vi "background writer.vi"(0 "dictionary":T1, 1 "command queue":refnum<k33>, 2 "response from processor":refnum<k33>, 3 "output type order":T3[](array[typedef]), 5 "logging path":path, 7 "backup directory":path, 9 "cache allocation":T2, 11 "scans per write":u16=20, 12 "group name":string, 13 "enable channel (bool)":i32, 14 "has enable channel":bool) -> (15 "error out":errorcluster)   [LabVIEW 2013, in "TDMS datalogger runtime.lvclass"]
uses:
  TDMS datalogger runtime.lvclass
  <vilib>/NI/Tag Bus/tag/Data Type.ctl
  data cache.ctl
  <vilib>/NI/Tag Bus/dictionary/full data dictionary.ctl
  message to background process.ctl
  control enum.ctl
  <vilib>/NI/Tag Bus/table/data table.ctl
  response from background process.ctl
  response enum.ctl
  writer state enum.ctl
  move to cache.vi
  write cache to tdms.vi
  <vilib>/NI/Tag Bus/table/data table.lvlib
  <vilib>/NI/Tag Bus/tag/tag descriptor.lvclass
  <vilib>/NI/Tag Bus/dictionary/data dictionary.lvclass
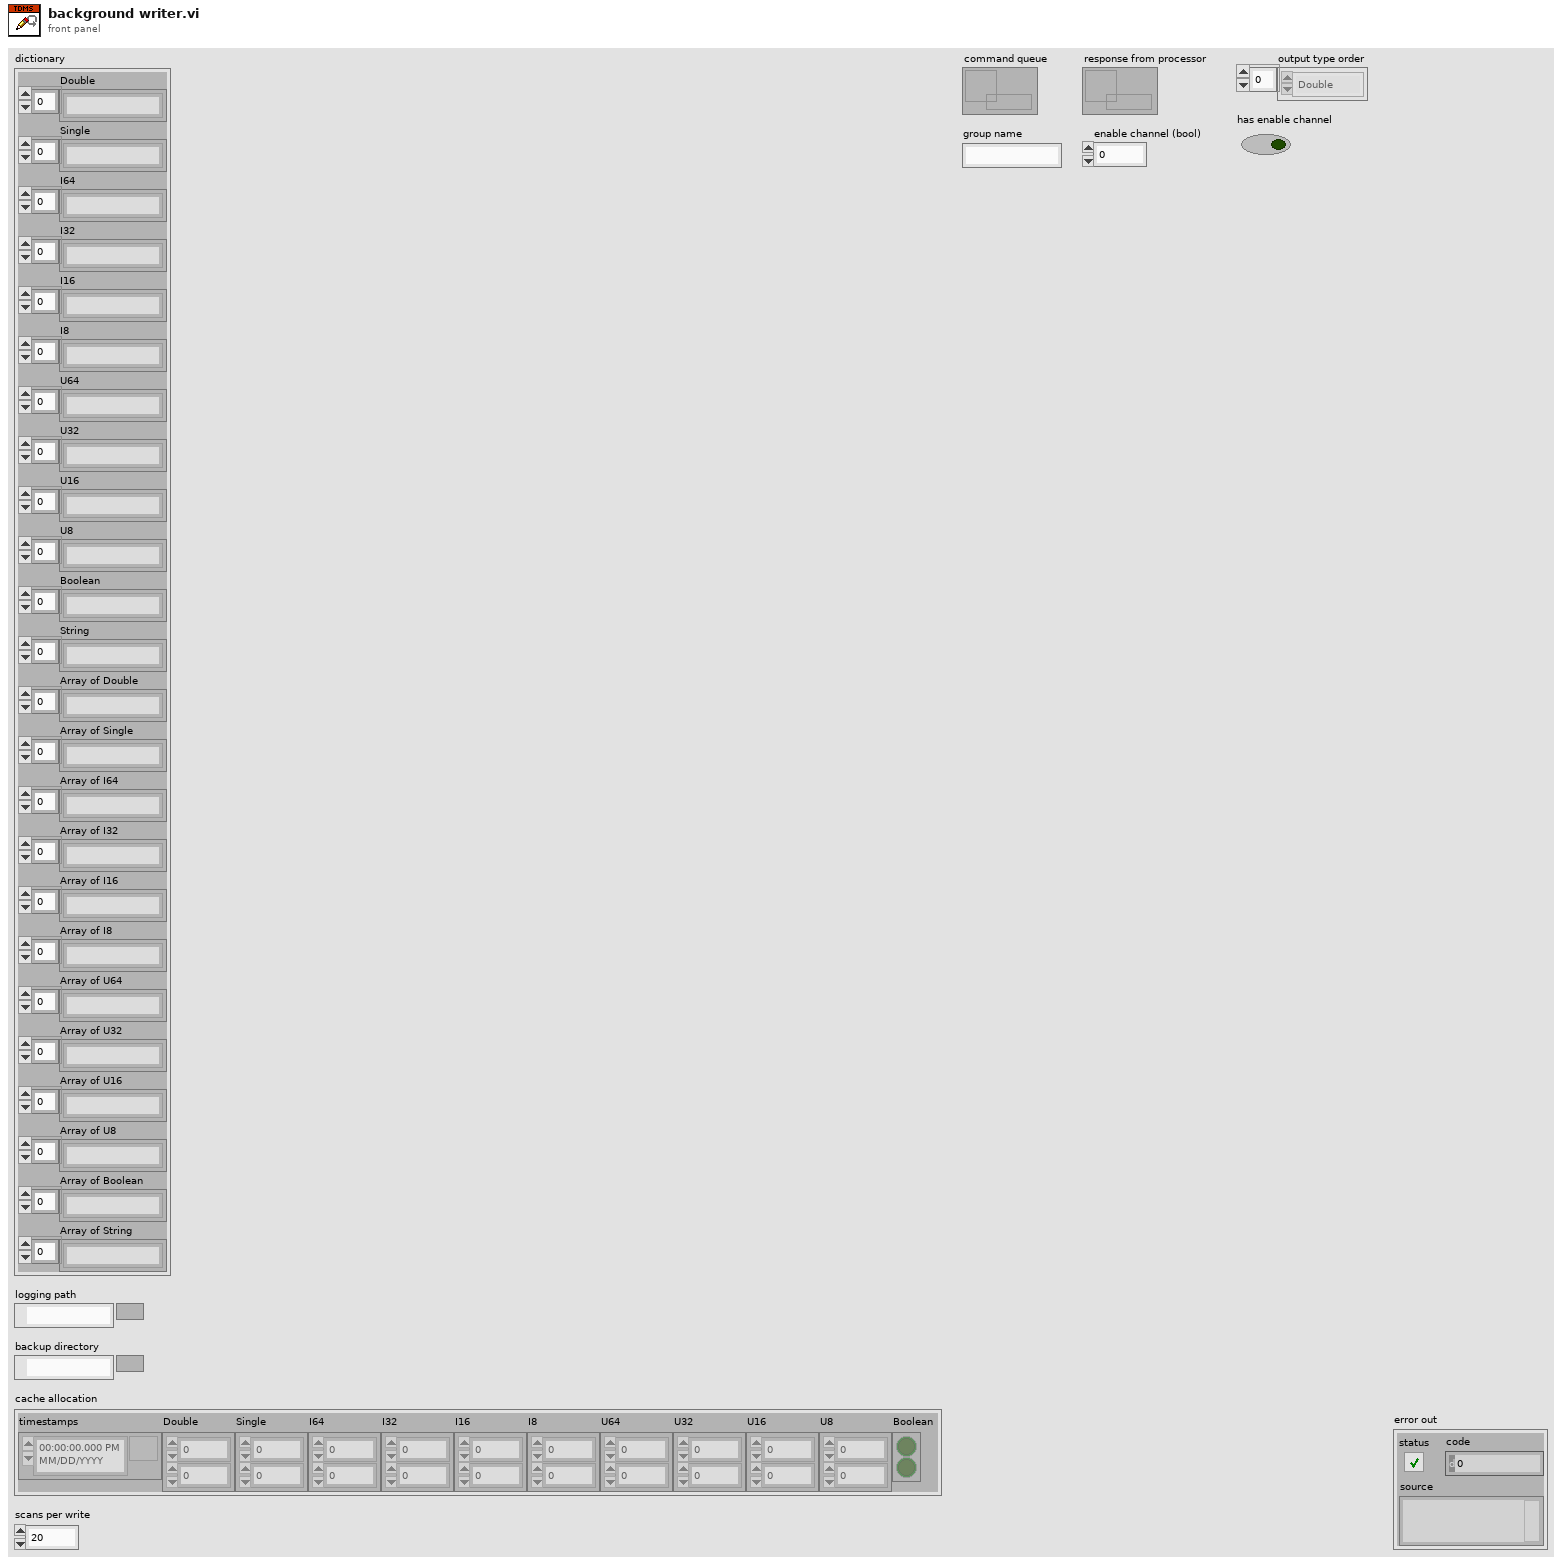
[diagram p1: front panel]
types:
  T1 = typedef "tag bus.lvlib/data dictionary.lvclass/full data dictionary.ctl" = cluster{"Double":string[], "Single":string[], "I64":string[], "I32":string[], "I16":string[], "I8":string[], "U64":string[], "U32":string[], "U16":string[], "U8":string[], "Boolean":string[], "String":string[], "Array of Double":string[], "Array of Single":string[], "Array of I64":string[], "Array of I32":string[], "Array of I16":string[], "Array of I8":string[], "Array of U64":string[], "Array of U32":string[], "Array of U16":string[], "Array of U8":string[], "Array of Boolean":string[], "Array of String":string[]}
  T2 = typedef "TDMS datalogger runtime.lvclass/data cache.ctl" = cluster{"timestamps":timestamp[], "Double":dbl[][], "Single":sgl[][], "I64":i64[][], "I32":i32[][], "I16":i16[][], "I8":i8[][], "U64":u64[][], "U32":u32[][], "U16":u16[][], "U8":u8[][], "Boolean":bool[][]}
  T3 = typedef "tag bus.lvlib/tag descriptor.lvclass/Data Type.ctl" = enum16{"Double", "Single", "I64", "I32", "I16", "I8", "U64", "U32", "U16", "U8", "Boolean", "String", "Array of Double", "Array of Single", "Array of I64", "Array of I32", "Array of I16", "Array of I8", "Array of U64", "Array of U32", "Array of U16", "Array of U8", "Array of Boolean", "Array of String"}
  T4 = typedef "TDMS datalogger runtime.lvclass/writer state enum.ctl" = enum16{"wait for message", "create file", "report error", "exit", "close file"}
  T5 = typedef "TDMS datalogger runtime.lvclass/response enum.ctl" = enum16{"exit", "return buffer", "error"}
  T6 = typedef "TDMS datalogger runtime.lvclass/response from background process.ctl" = cluster{"response enum":T5, "datapack":refnum<data-value>, "error code":i32}
  T7 = typedef "TDMS datalogger runtime.lvclass/message to background process.ctl" = cluster{"control enum":T8, "datapack":refnum<data-value>, "Time Stamp":timestamp}
  T8 = typedef "TDMS datalogger runtime.lvclass/control enum.ctl" = enum16{"exit", "output data"}
  T9 = typedef "tag bus.lvlib/data table.lvlib/data table.ctl" = cluster{"Double":dbl[], "Single":sgl[], "I64":i64[], "I32":i32[], "I16":i16[], "I8":i8[], "U64":u64[], "U32":u32[], "U16":u16[], "U8":u8[], "Boolean":bool[], "String":string[], "Array of Double":cluster{"DBL Array":dbl[]}[], "Array of Single":cluster{"SGL Array":sgl[]}[], "Array of I64":cluster{"I64 Array":i64[]}[], "Array of I32":cluster{"I32 Array":i32[]}[], "Array of I16":cluster{"I16 Array":i16[]}[], "Array of I8":cluster{"I8 Array":i8[]}[], "Array of U64":cluster{"U64 Array":u64[]}[], "Array of U32":cluster{"U32 Array":u32[]}[], "Array of U16":cluster{"U16 Array":u16[]}[], "Array of U8":cluster{"U8 Array":u8[]}[], "Array of Boolean":cluster{"Boolean Array":bool[]}[], "Array of String":cluster{"String Array":string[]}[]}
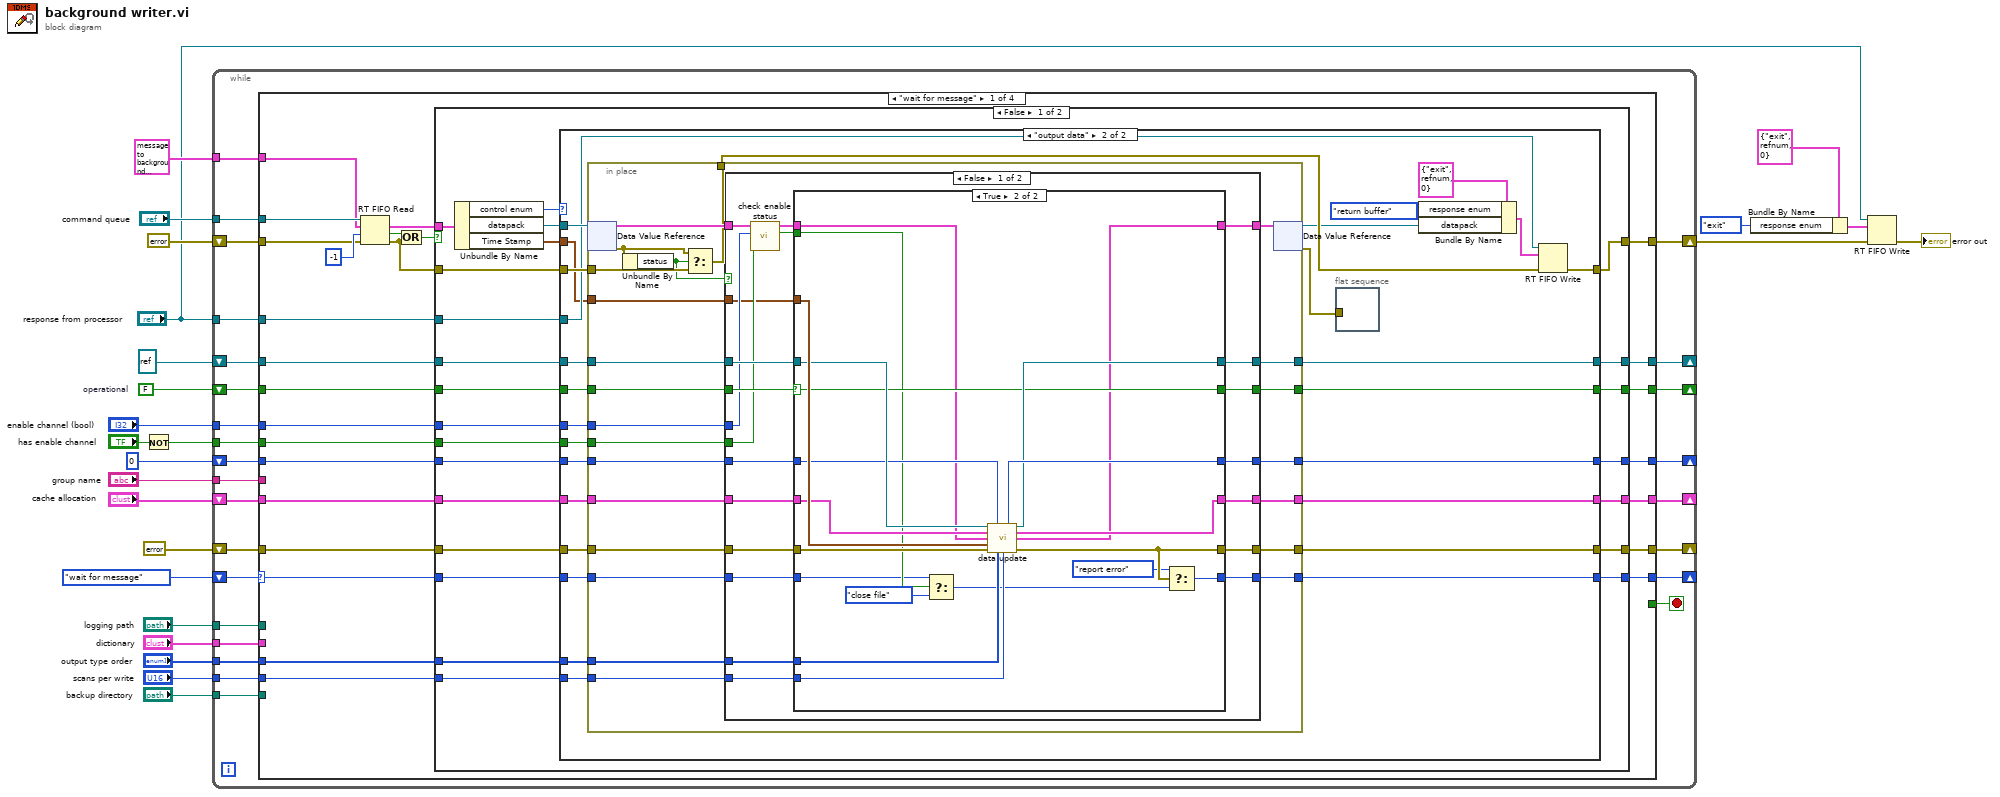
[diagram p0: block diagram]
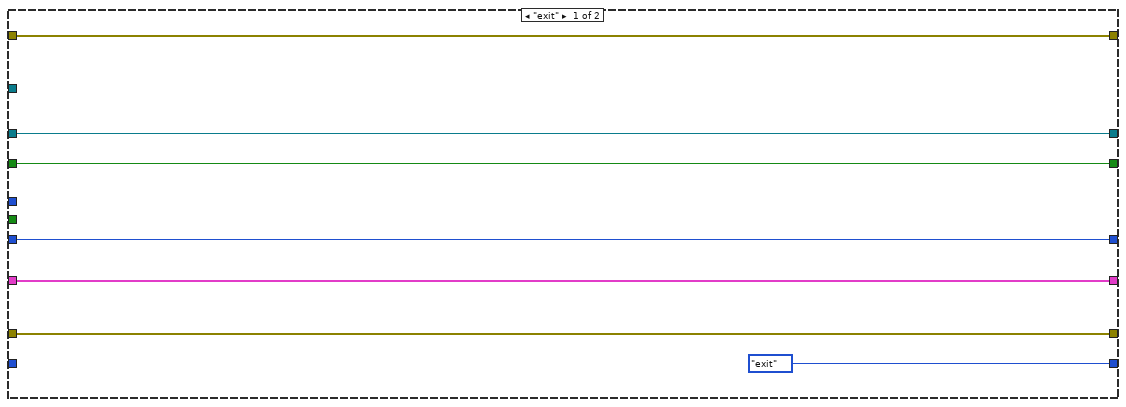
[diagram p2: hidden frame]
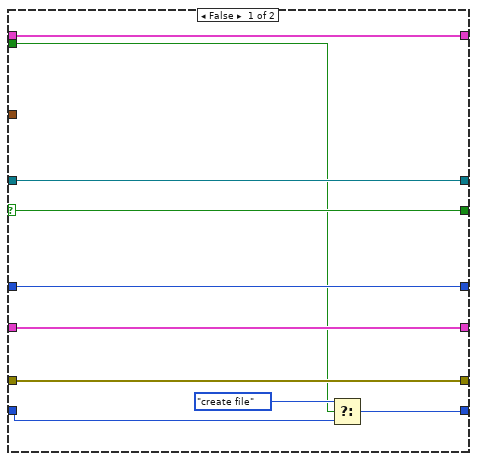
[diagram p3: hidden frame]
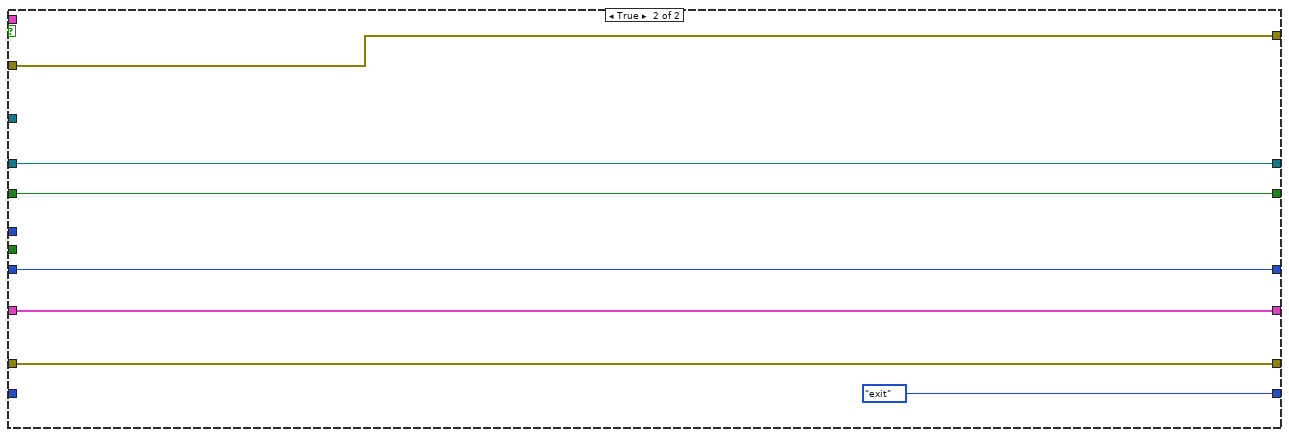
[diagram p5: hidden frame]
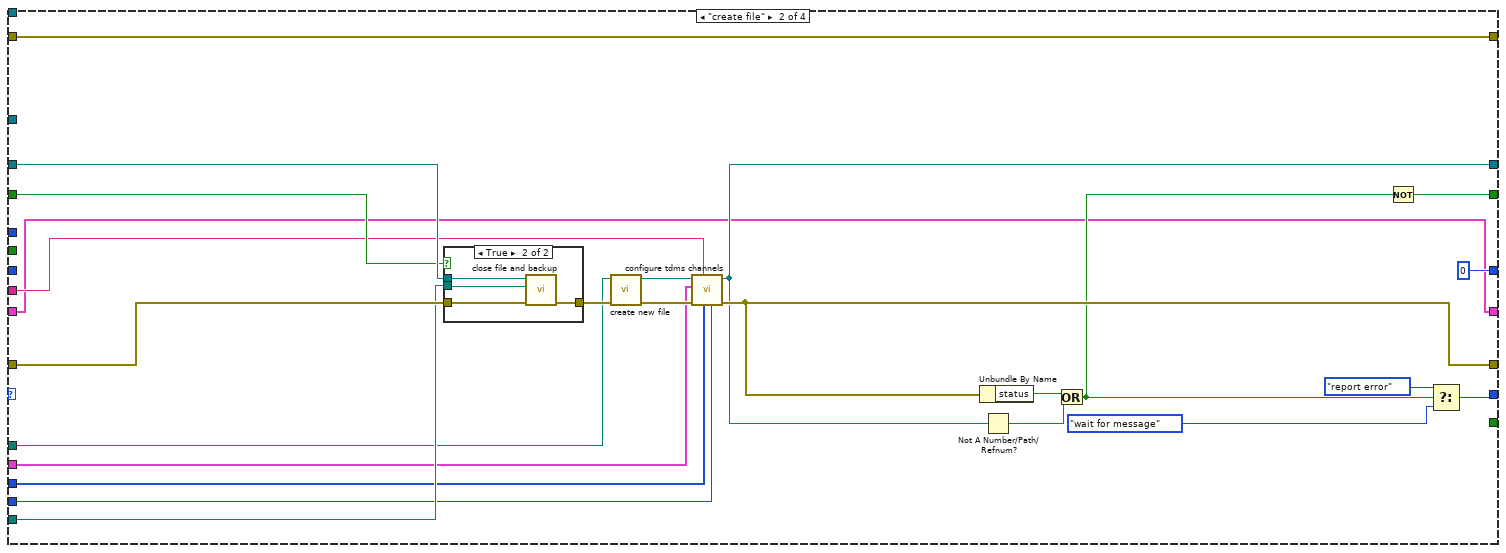
[diagram p6: hidden frame]
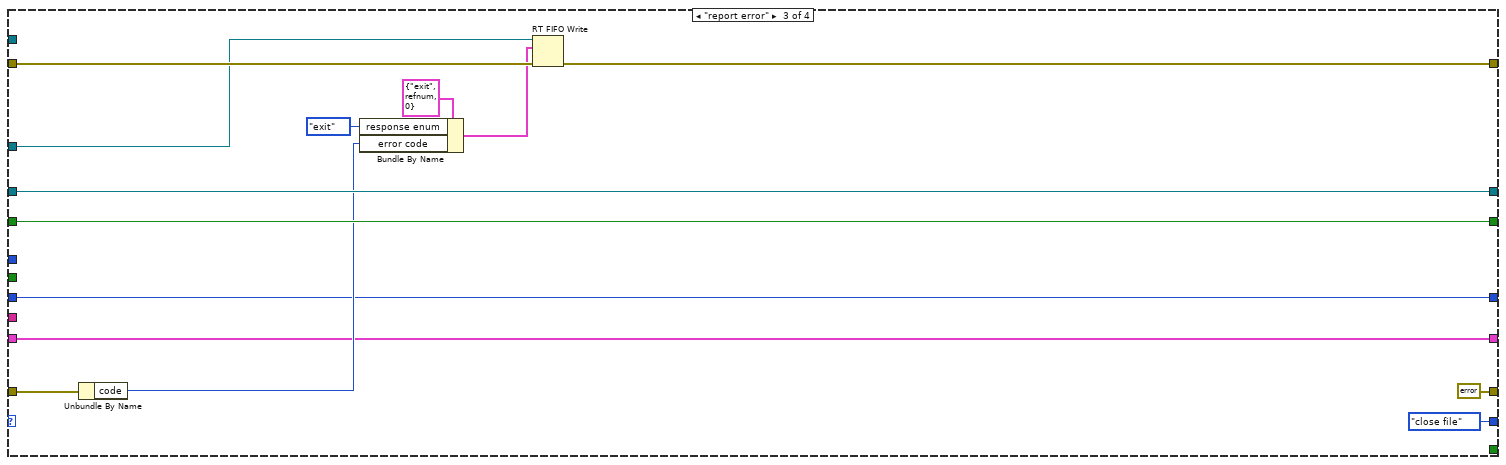
[diagram p8: hidden frame]
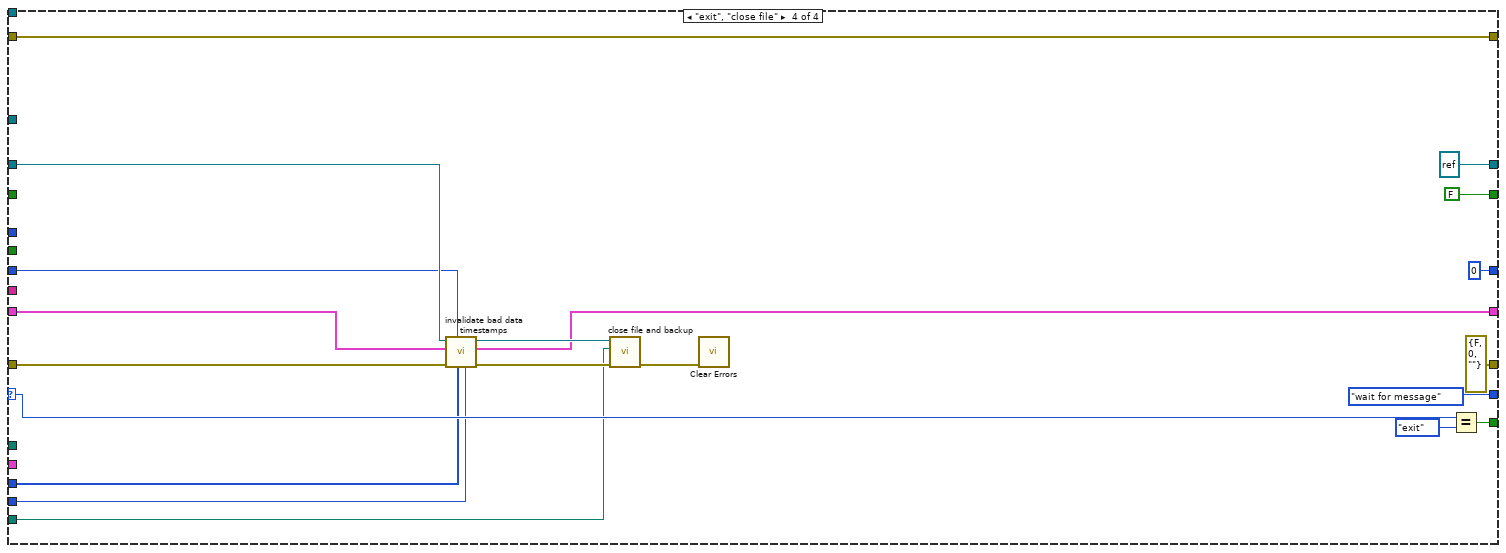
[diagram p9: hidden frame]
diagram:
  w13 = FALSE  # operational
  n1 = Not(x="has enable channel") -> (.not. x?=w5:bool)
  n2 = while {
    tunnel: "command queue" -> [w50]
    tunnel: T7 {"control enum"=enum."exit", "datapack"=refnum, "Time Stamp"=timestamp(0 s since 1904-01-01)} ("element") -> [w49]
    shift-right: [w47] -> w21
    shift-left: errorcluster {"status"=FALSE, "code"=0, "source"=""} ("error in") -> [w48]
    tunnel: "response from processor" -> [w45]
    shift-right: [w43] -> _
    shift-left: writer_state_enum."wait for message" ("logger state") -> [w44]
    shift-right: [w41] -> _
    shift-left: refnum<k34> refnum ("tdms file out") -> [w42]
    shift-right: [w32] -> _
    shift-left: w13 -> [w40]
    shift-right: [w38] -> _
    shift-left: errorcluster {"status"=FALSE, "code"=0, "source"=""} ("error in") -> [w39]
    tunnel: "logging path" -> [w37]
    tunnel: "dictionary" -> [w36]
    tunnel: "output type order" -> [w35]
    tunnel: "scans per write" -> [w34]
    tunnel: "backup directory" -> [w33]
    shift-right: [w31] -> _
    shift-left: 0 ("sample counter") -> [w30]
    shift-right: [w25] -> _
    shift-left: "cache allocation" -> [w26]
    tunnel: "enable channel (bool)" -> [w28]
    tunnel: w5 -> [w29]
    tunnel: "group name" -> [w27]
    stop <- w46 stop-if-true
    n3 = case shown="\"wait for message\"" w44 {
      selector: w44 -> [w55 _ _ w282]
      tunnel: w50 -> [w76 _ _ _]
      tunnel: w49 -> [w74 _ _ _]
      tunnel: w48 -> [w73 w226 w264 w284]
      tunnel: [w69 w226 w262 w284] -> w47
      tunnel: [_ _ _ w283] -> w46
      tunnel: w45 -> [w67 _ w261 _]
      tunnel: [w66 w230 writer_state_enum."close file" ("logger state") writer_state_enum."wait for message" ("logger state")] -> w43
      tunnel: w42 -> [w65 w238 w263 w276]
      tunnel: [w64 w227 w263 refnum<k34> refnum ("tdms file out")] -> w41
      tunnel: w40 -> [w62 w225 w255 _]
      tunnel: w39 -> [w60 w240 w254 w277]
      tunnel: [w61 w239 errorcluster {"status"=FALSE, "code"=0, "source"=""} ("error out") errorcluster {"status"=FALSE, "code"=0, "source"=""} ("error out")] -> w38
      tunnel: w37 -> [_ w236 _ _]
      tunnel: w36 -> [_ w235 _ _]
      tunnel: w35 -> [w52 w234 _ w270]
      tunnel: w34 -> [w51 w233 _ w269]
      tunnel: w33 -> [_ w237 _ w274]
      tunnel: [w63 w228 w255 FALSE] -> w32
      tunnel: [w58 0 ("sample counter") w251 0 ("sample counter")] -> w31
      tunnel: w30 -> [w59 _ w251 w271]
      tunnel: w29 -> [w53 _ _ _]
      tunnel: w28 -> [w54 _ _ _]
      tunnel: w27 -> [_ w223 _ _]
      tunnel: w26 -> [w57 w222 w252 w273]
      tunnel: [w56 w222 w252 w272] -> w25
      frame "wait for message" {
        n4 = RT FIFO Read(0:w76, 1:w74, 2:-1 ("timeout in ms (0)"), 3:w73) -> (9:w68:T7, 10:w72:bool, 11:w70:errorcluster)  [unwired: 2 out]
        n5 = Or(x=w72, y=w70) -> (x .or. y?=w71:bool)
        n6 = case shown="False" w71 {
          tunnel: w70 -> [w96 w221]
          tunnel: [w97 w221] -> w69
          tunnel: w68 -> [w99 _]
          tunnel: w67 -> [w93 _]
          tunnel: [w92 writer_state_enum."exit" ("logger state")] -> w66
          tunnel: w65 -> [w91 w219]
          tunnel: [w90 w219] -> w64
          tunnel: [w88 w218] -> w63
          tunnel: w62 -> [w89 w218]
          tunnel: [w87 w217] -> w61
          tunnel: w60 -> [w86 w217]
          tunnel: w59 -> [w84 w216]
          tunnel: [w85 w216] -> w58
          tunnel: w57 -> [w83 w215]
          tunnel: [w82 w215] -> w56
          tunnel: w55 -> [w81 _]
          tunnel: w54 -> [w80 _]
          tunnel: w53 -> [w79 _]
          tunnel: w52 -> [w78 _]
          tunnel: w51 -> [w77 _]
          frame False {
            n7 = Unbundle By Name(w99) -> ("control enum"=w98:T8, "datapack"=w94:refnum<data-value>, "Time Stamp"=w95:timestamp)
            n8 = case shown="\"output data\"" w98 {
              tunnel: [w106 w117] -> w97
              tunnel: w96 -> [w106 w132]
              tunnel: w95 -> [_ w109]
              tunnel: w94 -> [_ w133]
              tunnel: w93 -> [_ w114]
              tunnel: [writer_state_enum."exit" ("logger state") w121] -> w92
              tunnel: w91 -> [w104 w131]
              tunnel: [w104 w130] -> w90
              tunnel: w89 -> [w103 w128]
              tunnel: [w103 w129] -> w88
              tunnel: [w102 w122] -> w87
              tunnel: w86 -> [w102 w123]
              tunnel: [w100 w126] -> w85
              tunnel: w84 -> [w100 w127]
              tunnel: w83 -> [w101 w124]
              tunnel: [w101 w125] -> w82
              tunnel: w81 -> [_ w120]
              tunnel: w80 -> [_ w119]
              tunnel: w79 -> [_ w118]
              tunnel: w78 -> [_ w108]
              tunnel: w77 -> [_ w107]
              frame "exit" {
              }
              frame "output data" {
                n9 = in-place {
                  in-place-border: w132 -> [w156]
                  in-place-border: w131 -> [w151]
                  in-place-border: [w150] -> w130
                  in-place-border: [w149] -> w129
                  in-place-border: w128 -> [w148]
                  in-place-border: w127 -> [w147]
                  in-place-border: [w146] -> w126
                  in-place-border: [w145] -> w125
                  in-place-border: w124 -> [w144]
                  in-place-border: w123 -> [w143]
                  in-place-border: [w142] -> w122
                  in-place-border: [w141] -> w121
                  in-place-border: w120 -> [w140]
                  in-place-border: [w139] -> w116
                  in-place-border: w119 -> [w138]
                  in-place-border: w118 -> [w137]
                  in-place-border: w109 -> [w136]
                  in-place-border: w108 -> [w135]
                  in-place-border: w107 -> [w134]
                  n10 = in-place-dvr #1(w133) -> (w152:T9, w155:errorcluster)
                  n11 = Unbundle By Name(w155) -> ("status"=w154:bool)
                  n12 = Select(t=w155, s=w154, f=w156) -> (s? t:f=w139:errorcluster)
                  n13 = case shown="False" w154 {
                    tunnel: [w162 w214] -> w153
                    tunnel: w152 -> [w165 w214]
                    tunnel: w151 -> [w174 w213]
                    tunnel: [w175 w213] -> w150
                    tunnel: [w176 w212] -> w149
                    tunnel: w148 -> [w177 w212]
                    tunnel: w147 -> [w172 w211]
                    tunnel: [w173 w211] -> w146
                    tunnel: [w168 w210] -> w145
                    tunnel: w144 -> [w169 w210]
                    tunnel: w143 -> [w171 w209]
                    tunnel: [w170 w209] -> w142
                    tunnel: [w167 w208] -> w141
                    tunnel: w140 -> [w166 w208]
                    tunnel: w138 -> [w161 _]
                    tunnel: w137 -> [w160 _]
                    tunnel: w136 -> [w159 _]
                    tunnel: w135 -> [w158 _]
                    tunnel: w134 -> [w157 _]
                    frame False {
                      n14 = call "check enable status.vi"("always enabled?"=w160, "enable channel index"=w161, "data table in"=w165) -> ("enabled?"=w163:bool, "Data table out"=w164:T9)  [unwired: 7 in]
                      n15 = case shown="True" w177 {
                        selector: w177 -> [w187 w199]
                        tunnel: [w187 w199] -> w176
                        tunnel: [w186 w200] -> w175
                        tunnel: w174 -> [w186 w205]
                        tunnel: [w184 w202] -> w173
                        tunnel: w172 -> [w184 w203]
                        tunnel: w171 -> [w185 w207]
                        tunnel: [w185 w198] -> w170
                        tunnel: w169 -> [w183 w204]
                        tunnel: [w183 w201] -> w168
                        tunnel: [w182 w197] -> w167
                        tunnel: w166 -> [w180 w190]
                        tunnel: w164 -> [w178 w194]
                        tunnel: w163 -> [w179 w191]
                        tunnel: [w178 w195] -> w162
                        tunnel: w159 -> [_ w206]
                        tunnel: w158 -> [_ w193]
                        tunnel: w157 -> [_ w192]
                        frame False {
                          n16 = Select(t=writer_state_enum."create file" ("logger state"), s=w179, f=w180) -> (s? t:f=w182:T4)
                        }
                        frame True {
                          n17 = Select(t=w190, s=w191, f=writer_state_enum."close file") -> (s? t:f=w188:T4)
                          n18 = call "data update.vi"("tdms in"=w205, "sample counter in"=w203, "cache in"=w204, "data table in"=w194, "Time Stamp"=w206, "error in"=w207, "output type order"=w193, "scans per write"=w192) -> ("sample counter out"=w202:i32, "tdms out"=w200:refnum<k34>, "cache out"=w201:T2, "data table out"=w195:T9, "error out"=w198:errorcluster)  [unwired: 3 in]
                          n19 = Select(t=writer_state_enum."report error", s=w198, f=w188) -> (s? t:f=w197:T4)
                        }
                      }
                    }
                    frame True {
                    }
                  }
                  n20 = in-place-dvr #1(w153) -> (w111:refnum<data-value>, w115:errorcluster)
                }
                n21 = flat-sequence {
                  tunnel: w115 -> [_]
                  frame #0 {
                  }
                }
                n22 = Bundle By Name(cluster=T6 {"response enum"=enum."exit", "datapack"=refnum, "error code"=0} ("element"), "response enum"=response_enum."return buffer", "datapack"=w111) -> (w112:T6)
                n23 = RT FIFO Write(0:w114, 1:w112, 3:w116) -> (11:w117:errorcluster)  [unwired: 2 in, 3 out]
              }
            }
          }
          frame True {
          }
        }
      }
      frame "create file" {
        n24 = case shown="True" w225 {
          tunnel: [w246 w249] -> w241
          tunnel: w240 -> [w246 w250]
          tunnel: w238 -> [_ w248]
          tunnel: w237 -> [_ w247]
          frame False {
          }
          frame True {
            n25 = call "close file and backup.vi"("error in"=w250, "backup directory"=w247, "tdms file in"=w248) -> ("error out"=w249:errorcluster)  [unwired: 8 in]
          }
        }
        n26 = call "create new file.vi"("error in"=w241, "logging path"=w236) -> ("error out"=w242:errorcluster, "tdms file out"=w243:refnum<k34>)  [unwired: 8 in]
        n27 = call "configure tdms channels.vi"("samples per channel (1)"=w233, "type order"=w234, "group name"=w223, "error in"=w242, "dictionary"=w235, "tdms file in"=w243) -> ("error out"=w239:errorcluster, "tdms file out"=w227:refnum<k34>)  [unwired: 4 in]
        n28 = Unbundle By Name(w239) -> ("status"=w245:bool)
        n29 = Not A Number/Path/Refnum?(number/path/refnum=w227) -> (NaN/Path/Refnum?=w244:bool)
        n30 = Or(x=w245, y=w244) -> (x .or. y?=w229:bool)
        n31 = Not(x=w229) -> (.not. x?=w228:bool)
        n32 = Select(t=writer_state_enum."report error" ("logger state"), s=w229, f=writer_state_enum."wait for message" ("logger state")) -> (s? t:f=w230:T4)
      }
      frame "report error" {
        n33 = Unbundle By Name(w254) -> ("code"=w253:i32)
        n34 = Bundle By Name(cluster=T6 {"response enum"=enum."exit", "datapack"=refnum, "error code"=0} ("element"), "response enum"=response_enum."exit", "error code"=w253) -> (w259:T6)
        n35 = RT FIFO Write(0:w261, 1:w259, 3:w264) -> (11:w262:errorcluster)  [unwired: 2 in, 3 out]
      }
      frame "exit", "close file" {
        n36 = call "invalidate bad data timestamps.vi"("scans per write"=w269, "output type order"=w270, "sample counter"=w271, "error in"=w277, "cache allocation in"=w273, "tdms file in"=w276) -> ("error out"=w278:errorcluster, "cache allocation out"=w272:T2, "tdms file out"=w279:refnum<k34>)  [unwired: 3 in]
        n37 = call "close file and backup.vi"("error in"=w278, "backup directory"=w274, "tdms file in"=w279) -> ("error out"=w266:errorcluster)  [unwired: 8 in]
        n38 = call <vilib>:"Clear Errors.vi"("error in (no error)"=w266) -> ()  [unwired: 6 in, 1 out]
        n39 = Equal?(x=w282, y=writer_state_enum."exit") -> (x = y?=w283:bool)
      }
    }
  }
  n40 = Bundle By Name(cluster=T6 {"response enum"=enum."exit", "datapack"=refnum, "error code"=0} ("element"), "response enum"=response_enum."exit") -> (w18:T6)
  n41 = RT FIFO Write(0:"response from processor", 1:w18, 3:w21) -> (11:→"error out":errorcluster)  [unwired: 2 in, 3 out]
